vi "file read.vi"() -> ()   [LabVIEW 2020]
uses:
  file info.ctl
  track info.ctl
  event info.ctl
  event type.ctl
  midi file.lvclass
panel:
  out "Event Info":T1[][](array[typedef])
  out "Track Name":string[](array[string])
  out "Track Info":T3[](array[typedef])
  out "File Info":T4
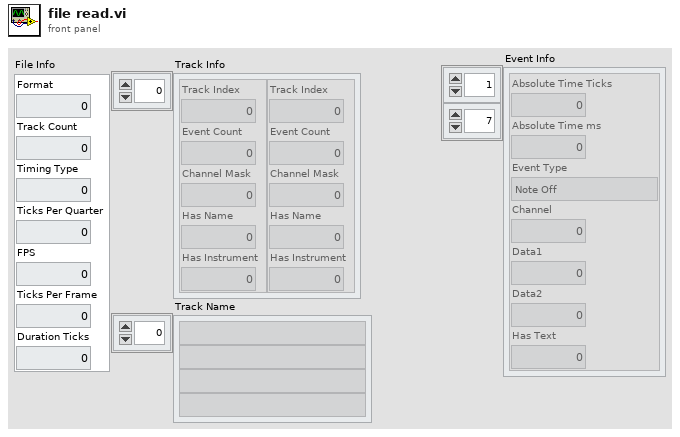
[diagram p1: front panel]
types:
  T1 = typedef "MIDIllan.lvlib/midi file.lvclass/event info.ctl" = cluster{"Absolute Time Ticks":u32, "Absolute Time ms":dbl, "Event Type":T2, "Channel":u8, "Data1":u8, "Data2":u8, "Has Text":i32}
  T2 = typedef "MIDIllan.lvlib/midi file.lvclass/event type.ctl" = enum32{"Note Off", "Note On", "Polyphonic Aftertouch", "Control Change", "Program Change", "Channel Aftertouch", "Pitch Bend", "System Exclusive", "8 - undefined", "9 - undefined", "10 - undefined", "11 - undefined", "12 - undefined", "13 - undefined", "14 - undefined", "15 - undefined", "16 - undefined", "17 - undefined", "18 - undefined", "19 - undefined", "20 - undefined", "21 - undefined", "22 - undefined", "23 - undefined", "24 - undefined", "25 - undefined", "26 - undefined", "27 - undefined", "28 - undefined", "29 - undefined", "30 - undefined", "31 - undefined", "32 - undefined", "33 - undefined", "34 - undefined", "35 - undefined", "36 - undefined", "37 - undefined", "38 - undefined", "39 - undefined", "40 - undefined", "41 - undefined", "42 - undefined", "43 - undefined", "44 - undefined", "45 - undefined", "46 - undefined", "47 - undefined", "48 - undefined", "49 - undefined", "50 - undefined", "51 - undefined", "52 - undefined", "53 - undefined", "54 - undefined", "55 - undefined", "56 - undefined", "57 - undefined", "58 - undefined", "59 - undefined", "60 - undefined", "61 - undefined", "62 - undefined", "63 - undefined", "64 - undefined", "65 - undefined", "66 - undefined", "67 - undefined", "68 - undefined", "69 - undefined", "70 - undefined", "71 - undefined", "72 - undefined", "73 - undefined", "74 - undefined", "75 - undefined", "76 - undefined", "77 - undefined", "78 - undefined", "79 - undefined", "80 - undefined", "81 - undefined", "82 - undefined", "83 - undefined", "84 - undefined", "85 - undefined", "86 - undefined", "87 - undefined", "88 - undefined", "89 - undefined", "90 - undefined", "91 - undefined", "92 - undefined", "93 - undefined", "94 - undefined", "95 - undefined", "96 - undefined", "97 - undefined", "98 - undefined", "99 - undefined", "Meta: Sequence Number", "Meta: Text", "Meta: Copyright", "Meta: Track Name", "Meta: Instrument Name", "Meta: Lyric", "Meta: Marker", "Meta: Cue Point", "Meta: Channel Prefix", "Meta: End of Track", "Meta: Set Tempo", "Meta: SMPTE Offset", "Meta: Time Signature", "Meta: Key Signature", "Meta: Sequencer Specific", "115 - undefined", "116 - undefined", "117 - undefined", "118 - undefined", "119 - undefined", "120 - undefined", "121 - undefined", "122 - undefined", "123 - undefined", "124 - undefined", "125 - undefined", "126 - undefined", "127 - undefined", "128 - undefined", "129 - undefined", "130 - undefined", "131 - undefined", "132 - undefined", "133 - undefined", "134 - undefined", "135 - undefined", "136 - undefined", "137 - undefined", "138 - undefined", "139 - undefined", "140 - undefined", "141 - undefined", "142 - undefined", "143 - undefined", "144 - undefined", "145 - undefined", "146 - undefined", "147 - undefined", "148 - undefined", "149 - undefined", "150 - undefined", "151 - undefined", "152 - undefined", "153 - undefined", "154 - undefined", "155 - undefined", "156 - undefined", "157 - undefined", "158 - undefined", "159 - undefined", "160 - undefined", "161 - undefined", "162 - undefined", "163 - undefined", "164 - undefined", "165 - undefined", "166 - undefined", "167 - undefined", "168 - undefined", "169 - undefined", "170 - undefined", "171 - undefined", "172 - undefined", "173 - undefined", "174 - undefined", "175 - undefined", "176 - undefined", "177 - undefined", "178 - undefined", "179 - undefined", "180 - undefined", "181 - undefined", "182 - undefined", "183 - undefined", "184 - undefined", "185 - undefined", "186 - undefined", "187 - undefined", "188 - undefined", "189 - undefined", "190 - undefined", "191 - undefined", "192 - undefined", "193 - undefined", "194 - undefined", "195 - undefined", "196 - undefined", "197 - undefined", "198 - undefined", "199 - undefined", "200 - undefined", "201 - undefined", "202 - undefined", "203 - undefined", "204 - undefined", "205 - undefined", "206 - undefined", "207 - undefined", "208 - undefined", "209 - undefined", "210 - undefined", "211 - undefined", "212 - undefined", "213 - undefined", "214 - undefined", "215 - undefined", "216 - undefined", "217 - undefined", "218 - undefined", "219 - undefined", "220 - undefined", "221 - undefined", "222 - undefined", "223 - undefined", "224 - undefined", "225 - undefined", "226 - undefined", "227 - undefined", "228 - undefined", "229 - undefined", "230 - undefined", "231 - undefined", "232 - undefined", "233 - undefined", "234 - undefined", "235 - undefined", "236 - undefined", "237 - undefined", "238 - undefined", "239 - undefined", "240 - undefined", "241 - undefined", "242 - undefined", "243 - undefined", "244 - undefined", "245 - undefined", "246 - undefined", "247 - undefined", "248 - undefined", "249 - undefined", "250 - undefined", "251 - undefined", "252 - undefined", "253 - undefined", "254 - undefined", "Unknown"}
  T3 = typedef "MIDIllan.lvlib/midi file.lvclass/track info.ctl" = cluster{"Track Index":i32, "Event Count":i32, "Channel Mask":i32, "Has Name":i32, "Has Instrument":i32}
  T4 = typedef "MIDIllan.lvlib/midi file.lvclass/file info.ctl" = cluster{"Format":i32, "Track Count":i32, "Timing Type":i32, "Ticks Per Quarter":i32, "FPS":sgl, "Ticks Per Frame":i32, "Duration Ticks":u32}
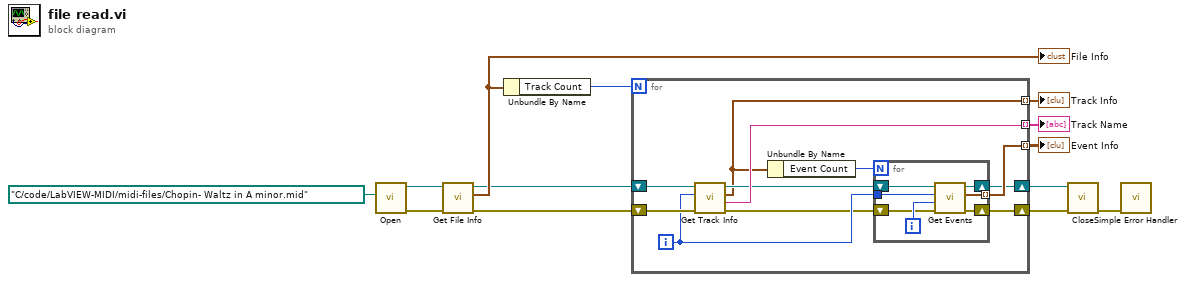
[diagram p0: block diagram]
diagram:
  n1 = call "Open.vi"("MIDI File"=path "C:/code/LabVIEW-MIDI/midi-files/Chopin- Waltz in A minor.mid") -> ("error out"=w10:errorcluster, "midi file"=w11:refnum<class "midi file.lvclass">)  [unwired: 9 in]
  n2 = call "Get File Info.vi"("error in (no error)"=w10, "midi file in"=w11) -> ("error out"=w8:errorcluster, "File Info"=w9:T4, "midi file out"=w6:refnum<class "midi file.lvclass">)  [unwired: 7 in]
  "File Info" <- w9
  n3 = Unbundle By Name(w9) -> ("Track Count"=w4:i32)
  n4 = for {
    N: w4 -> [_]
    shift-right: [w14] -> w7
    shift-left: w8 -> [w23]
    shift-right: [w16] -> w5
    shift-left: w6 -> [w24]
    tunnel: [w20] -> w3 mode=indexing
    tunnel: [w22] -> w2 mode=indexing
    tunnel: [w17] -> w1 mode=indexing
    i -> [w18]
    n5 = call "Get Track Info.vi"("error in (no error)"=w23, "Track Index"=w18, "midi file in"=w24) -> ("error out"=w15:errorcluster, "Track Name"=w22:string, "Track Info"=w20:T3, "midi file out"=w21:refnum<class "midi file.lvclass">)  [unwired: 5 in]
    n6 = Unbundle By Name(w20) -> ("Event Count"=w19:i32)
    n7 = for {
      N: w19 -> [_]
      tunnel: w18 -> [w30]
      tunnel: [w27] -> w17 mode=indexing
      shift-right: [w28] -> w16
      shift-left: w21 -> [w31]
      shift-right: [w26] -> w14
      shift-left: w15 -> [w25]
      i -> [w29]
      n8 = call "Get Events.vi"("error in (no error)"=w25, "Event Index"=w29, "Track Index"=w30, "midi file in"=w31) -> ("error out"=w26:errorcluster, "Event Details"=w27:T1, "midi file out"=w28:refnum<class "midi file.lvclass">)  [unwired: 5 in]
    }
  }
  "Track Info" <- w3
  "Track Name" <- w2
  "Event Info" <- w1
  n9 = call "Close.vi"("error in (no error)"=w7, "midi file"=w5) -> ("error out"=w13:errorcluster)  [unwired: 9 in]
  n10 = call <vilib>:"Simple Error Handler.vi"("error in (no error)"=w13) -> ()  [unwired: 4 in, 5 out]
